vi "题目3.vi"() -> ()   [LabVIEW 2017]
uses:
  <vilib>/measure/NI_MABase.lvlib
panel:
  out "Y":dbl[](array[numeric])
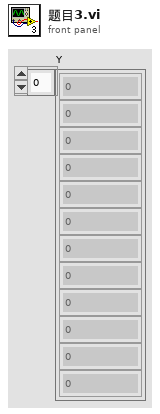
[diagram p1: front panel]
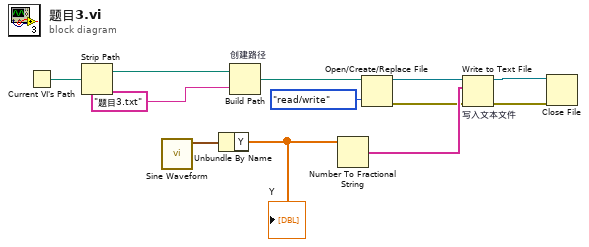
[diagram p0: block diagram]
diagram:
  n1 = Current VI's Path() -> (path=w11:path)
  n2 = Strip Path(path=w11) -> (stripped path=w10:path)  [unwired: 1 out]
  n3 = call <vilib>:"Sine Waveform.vi"() -> ("signal out"=w12:waveform(dbl))  [unwired: 10 in, 1 out]
  n4 = Unbundle By Name(w12) -> ("Y"=w5:dbl[])
  "Y" <- w5
  n5 = Build Path "创建路径"(base path=w10, name or relative path="题目3.txt" ("名称或相对路径")) -> (appended path=w8:path)
  n6 = Number To Fractional String(number=w5) -> (F-format string=w4:string[])  [unwired: 3 in]
  n7 = Open/Create/Replace File(file path (use dialog)=w8, access (0:read/write)=enum16{"read/write", "read-only", "write-only"}."read/write" ("权限(0:read/write)")) -> (refnum out=w6:refnum<file>, error out=w1:errorcluster)  [unwired: 4 in, 1 out]
  n8 = Write to Text File "写入文本文件"(file (use dialog)=w6, text=w4, error in=w1) -> (refnum out=w3:refnum<file>, error out=w2:errorcluster)  [unwired: 1 in, 1 out]
  n9 = Close File(refnum=w3, error in=w2) -> ()  [unwired: 2 out]
